vi "Shutdown Daemon.vi"(8 "error in (no error)":errorcluster, 11 "network slave in":refnum<class "Network Slave.lvclass">) -> (0 "error out":errorcluster)   [LabVIEW 2018, in "SubVIs.lvlib" / "Network Slave.lvclass"]
doc: "This provides an interface for the slave to shut down its protocol daemon."
uses:
  Network Slave.lvclass
  Network Slave.lvclass/Network Slave.ctl
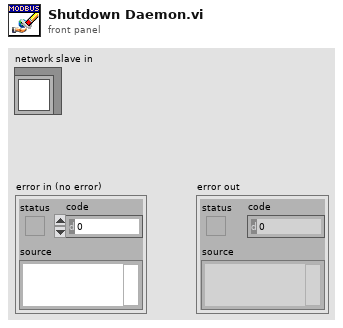
[diagram p1: front panel]
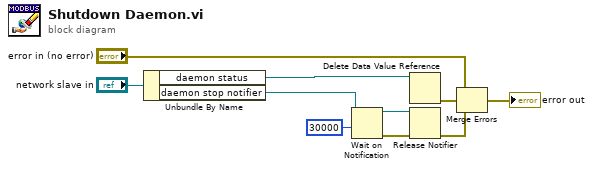
[diagram p0: block diagram]
diagram:
  n1 = Unbundle By Name("network slave in") -> ("daemon status"=w9:refnum<data-value>, "daemon stop notifier"=w5:refnum<notifier>)
  n2 = Wait on Notification(notifier=w5, timeout in ms (-1)=30000) -> (notifier out=w1:refnum<notifier>, error out=w3:errorcluster)  [unwired: 2 in, 2 out]
  n3 = Delete Data Value Reference(data value reference=w9) -> (error out=w8:errorcluster)  [unwired: 1 in, 1 out]
  n4 = Release Notifier(notifier=w1, error in (no error)=w3) -> (error out=w2:errorcluster)  [unwired: 1 in, 2 out]
  n5 = Merge Errors("error in (no error)", w8, w2) -> (→"error out":errorcluster)
